vi "Filter DependentTypeDefs&Parents.vi"(9 "Parent VI Name":string, 10 "Dependency Name":string, 11 "Dependendent TypeDefs wParents (in)":T1[](array[typedef])) -> (3 "Dependendent TypeDefs wParents (out)":T1[](array[typedef]))   [LabVIEW 2013, in "DiscoverCommonTypeDefCallers.lvlib"]
uses:
  DiscoverCommonTypeDefCallers.lvlib
  DependendentTypeDefwParents.ctl
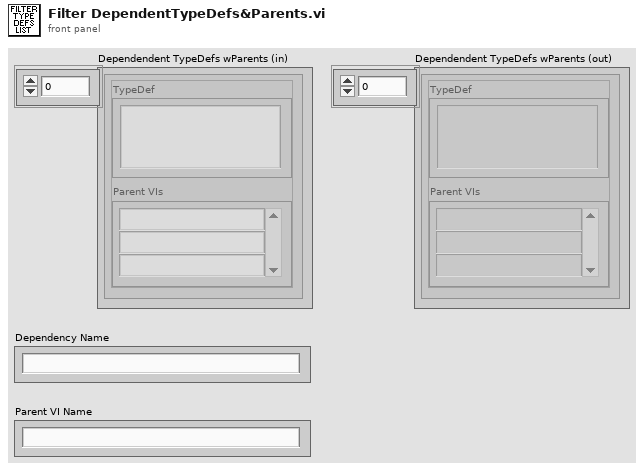
[diagram p1: front panel]
types:
  T1 = typedef "DiscoverCommonTypeDefCallers.lvlib/DependendentTypeDefwParents.ctl" = cluster{"TypeDef":string, "Parent VIs":string[]}
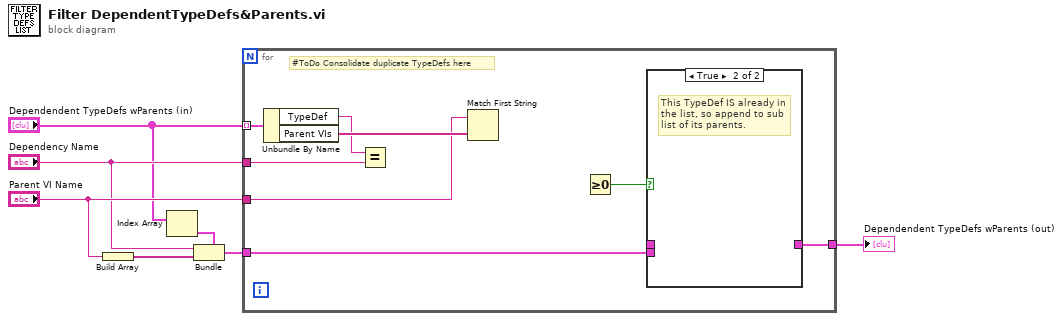
[diagram p0: block diagram]
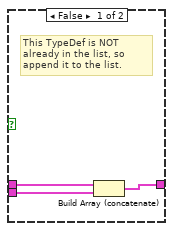
[diagram p2: hidden frame]
diagram:
  n1 = Build Array("Parent VI Name") -> (w6:string[])
  n2 = Index Array(array="Dependendent TypeDefs wParents (in)") -> (element=w7:T1)  [unwired: 1 in]
  n3 = Bundle(cluster=w7, "TypeDef"="Dependency Name", "Parent VIs"=w6) -> (w2:T1)
  n4 = for {
    tunnel: "Dependendent TypeDefs wParents (in)" -> [w15] mode=indexing
    tunnel: "Parent VI Name" -> [w13]
    tunnel: "Dependency Name" -> [w12]
    tunnel: w2 -> [w8]
    tunnel: [w9] -> w1
    # "#ToDo Consolidate duplicate TypeDefs here"
    n5 = Unbundle By Name(w15) -> ("TypeDef"=w11:string, "Parent VIs"=w14:string[])
    n6 = Equal?(x=w11, y=w12) -> ()  [unwired: 1 out]
    n7 = Match First String(2:w14, 3:w13) -> ()  [unwired: 2 out]
    n8 = Greater Or Equal To 0?() -> (x >= 0?=w10:bool)  [unwired: 1 in]
    n9 = case shown="True" w10 {
      tunnel: _ -> [w17 _]
      tunnel: [w18 _] -> w9
      tunnel: w8 -> [w16 _]
      frame False {
        # "This TypeDef is NOT already in the list, so append it to the list."
        n10 = Build Array (concatenate)(w17, w16) -> (w18:T1[])
      }
      frame True {
        # "This TypeDef IS already in the list, so append to sub list of its parents."
      }
    }
  }
  "Dependendent TypeDefs wParents (out)" <- w1
